vi "RFH-read_folder-common_format.vi"(0 "error out":errorcluster, 7 "Folder Path":path) -> (1 "Data":T1[](array[typedef]), 2 "Names":string[](array[string]))   [LabVIEW 2020, in "RFH-Reflection_File_Handler.lvlib"]
uses:
  RFH-Reflection_File_Handler.lvlib
  RFH-common_data_format.ctl
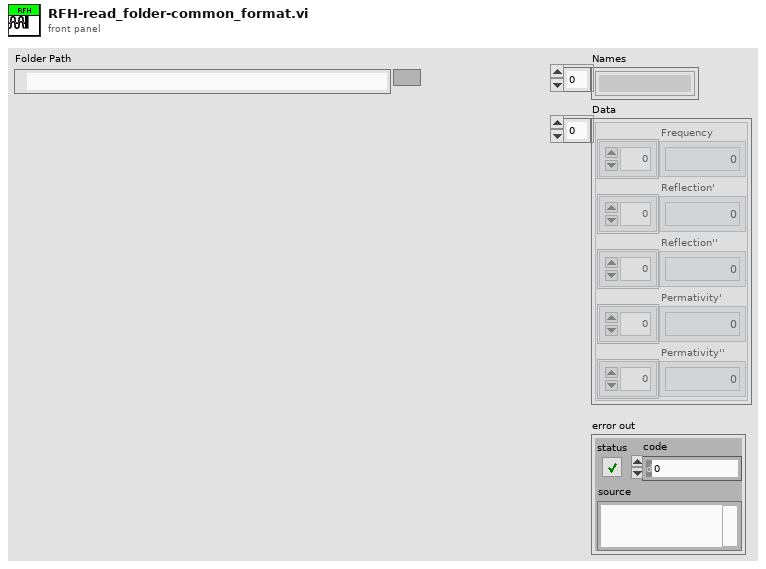
[diagram p1: front panel]
types:
  T1 = typedef "RFH-Reflection_File_Handler.lvlib/RFH-common_data_format.ctl" = cluster{"Frequency":dbl[], "Reflection'":dbl[], "Reflection''":dbl[], "Permativity'":dbl[], "Permativity''":dbl[]}
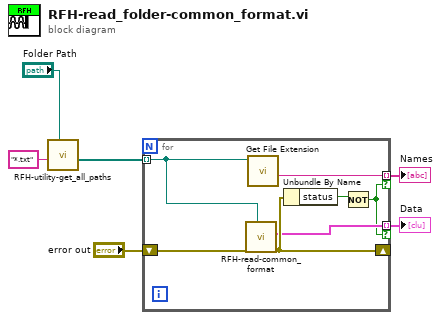
[diagram p0: block diagram]
diagram:
  n1 = call "RFH-utility-get_all_paths.vi"("Folder Path"="Folder Path", "pattern"="*.txt") -> ("All Files in Dir"=w6:path[])  [unwired: 6 in, 3 out]
  n2 = for {
    tunnel: w6 -> [w12] mode=indexing
    tunnel: [w13] -> w2 mode=indexing if=w7
    shift-right: [w10] -> _
    shift-left: "error out" -> [w11]
    tunnel: [w8] -> w1 mode=indexing if=w7
    n3 = call "RFH-read-common_format.vi"("file path (dialog if empty)"=w12, "error in"=w11) -> ("error out"=w10:errorcluster, "Common Format"=w8:T1)  [unwired: 8 in]
    n4 = call <vilib>:"Get File Extension.vi"("file"=w12) -> ("filename without extension"=w13:string)  [unwired: 6 in, 4 out]
    n5 = Unbundle By Name(w10) -> ("status"=w9:bool)
    n6 = Not(x=w9) -> (.not. x?=w7:bool)
  }
  "Names" <- w2
  "Data" <- w1
